vi "DisconnectAll.vi"(0 "reference in":refnum<class "Switch_Manager.lvclass">, 5 "error in (no error)":errorcluster) -> (14 "reference in":refnum<class "Switch_Manager.lvclass">, 19 "error out":errorcluster)   [LabVIEW 2022 SP3, in "Switch_Manager.lvlib" / "Switch_Manager.lvclass"]
uses:
  Switch_Manager.lvclass
  Components/SwitchBase.lvlibp/SwitchBase.lvclass
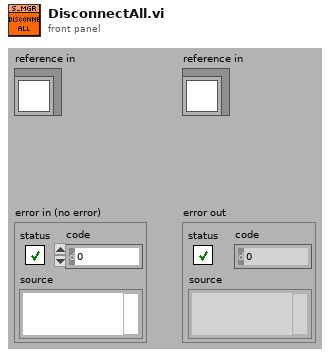
[diagram p1: front panel]
types:
  T1 = typedef "Switch_Manager.lvlib/Switch_Manager.lvclass/ObjectAttributes.ctl" = cluster{"Config":T2, "State":bool[], "Switches":refnum<class "SwitchBase.lvclass">[], "SwitchName":string[], "SwitchMap":T3[], "UpdateEvent":refnum<user-event>, "ParentEvent":refnum<user-event>, "Tree":bool[]}
  T2 = typedef "Switch_Manager.lvlib/Switch_Manager.lvclass/Config.ctl" = cluster{"default":string}
  T3 = typedef "Switch_Manager.lvlib/Switch_Manager.lvclass/SwitchMap.ctl" = cluster{"Name":string, "Description":string, "Group":string, "IsGroup":bool, "Switches":string[]}
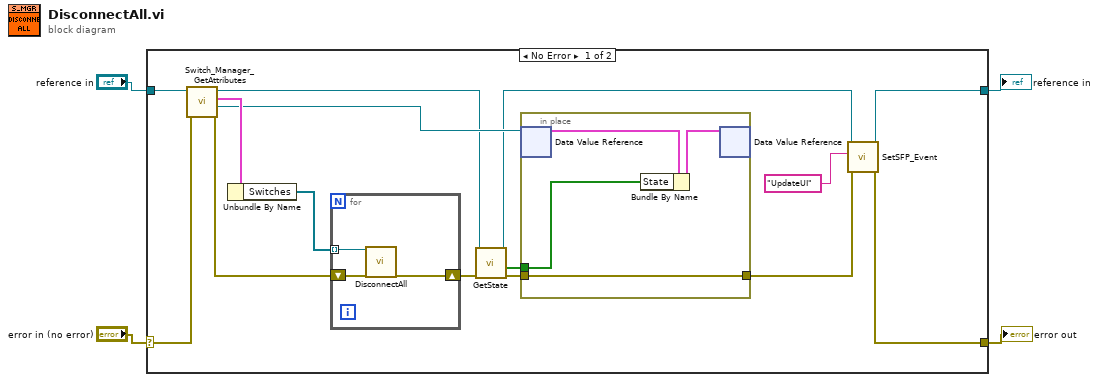
[diagram p0: block diagram]
diagram:
  n1 = case shown="No Error" "error in (no error)" {
    selector: "error in (no error)" -> [w19 w28]
    tunnel: [w13 w28] -> w3
    tunnel: [w11 w27] -> w1
    tunnel: "reference in" -> [w17 w27]
    frame No Error {
      n2 = call "Switch_Manager_GetAttributes.vi"("error in (no error)"=w19, "reference in"=w17) -> ("error out"=w16:errorcluster, "DataRef"=w15:refnum<data-value>, "Data"=w18:T1, "reference out"=w7:refnum<class "Switch_Manager.lvclass">)  [unwired: 6 in]
      n3 = Unbundle By Name(w18) -> ("Switches"=w10:refnum<class "SwitchBase.lvclass">[])
      n4 = for {
        shift-right: [w21] -> w9
        shift-left: w16 -> [w22]
        tunnel: w10 -> [w20] mode=indexing
        n5 = call-dynamic "DisconnectAll.vi"("reference in"=w20, "error in (no error)"=w22) -> ("error out"=w21:errorcluster)  [unwired: 16 in, 1 out]
      }
      n6 = call-dynamic "GetState.vi"("error in (no error)"=w9, "reference in"=w7) -> ("error out"=w8:errorcluster, "States"=w5:bool[], "reference in"=w6:refnum<class "Switch_Manager.lvclass">)  [unwired: 6 in, 1 out]
      n7 = in-place {
        in-place-border: w8 -> [w26]
        in-place-border: [w26] -> w12
        in-place-border: w5 -> [w23]
        n8 = in-place-dvr #1(w15) -> (w25:T1)  [unwired: 1 out]
        n9 = Bundle By Name(cluster=w25, "State"=w23) -> (w24:T1)
        n10 = in-place-dvr #1(w24) -> ()  [unwired: 2 out]
      }
      n11 = call-dynamic "SetSFP_Event.vi"("error in (no error)"=w12, "msg"="UpdateUI", "reference in"=w6) -> ("error out"=w13:errorcluster, "reference out"=w11:refnum<class "Switch_Manager.lvclass">)  [unwired: 7 in]
    }
    frame Error {
    }
  }
  "error out" <- w3
  "reference in" <- w1
